vi "ValFromATR(SubVI).vi"(8 "error in (no error)":errorcluster, 10 "Row":i32, 11 "Table in":refnum<vi>) -> (0 "error out":errorcluster, 3 "Val":dbl)   [LabVIEW 2017]
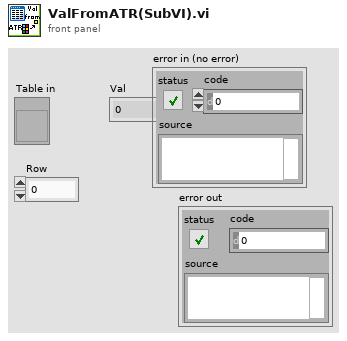
[diagram p1: front panel]
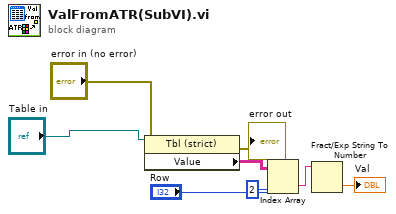
[diagram p0: block diagram]
diagram:
  n1 = property class="Tbl (strict)"(reference="Table in", error in="error in (no error)") -> (error out=→"error out":errorcluster, "Value"=w4:string[][])  [unwired: 1 out]
  n2 = Index Array(array=w4, index (row)="Row", index (col)=2 ("disabled index (col)")) -> (element=w7:string)
  n3 = Fract/Exp String To Number(string=w7) -> (number=→"Val":dbl)  [unwired: 3 in, 1 out]
